vi "PH_ImageStatistician.select Data.vi"(6 "Data Selector":T2 items=["nothing ", "FWHM Major Trace", "FWHM Minor Trace", "Gaussian Fit Order Major Trace", "Gaussian Fit Order Minor Trace", "99% Diameter Major Trace", "99% Diameter Minor Trace", "Theta", "Delta", "Major Diameter", "Minor Diameter", "Azimuth Angle", "Azi Angle rel to Major?", "Ellipticity", "Center of gravity - x", "Center of gravity - y", "Energy"], 8 "Statistician Data":T1) -> (1 "Data chosen?":bool, 2 "Data Legend":string, 3 "Data":dbl)   [LabVIEW 2014, in "PH_ImageStatistician.lvlib"]
doc: "This VI selects the data to be indicated."
uses:
  PH_ImageStatistician.lvlib
  PH_ImageStatistician.select Data.ctl
  PH_ImageStatistician.Statistician Data.ctl
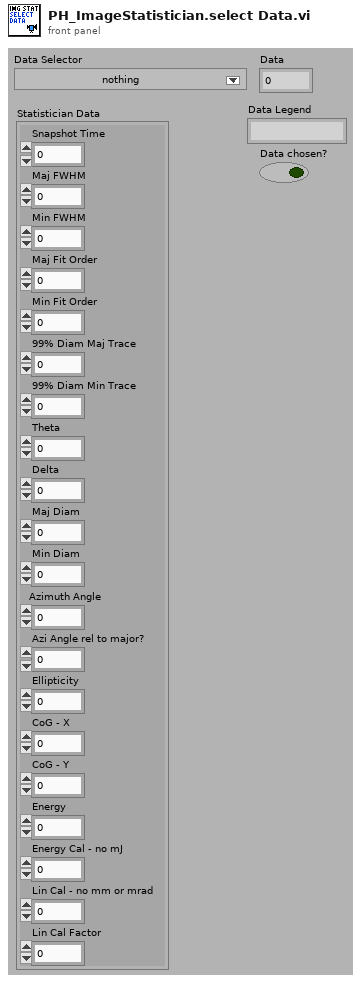
[diagram p1: front panel]
types:
  T1 = typedef "PH_ImageStatistician.lvlib/PH_ImageStatistician.Statistician Data.ctl" = cluster{"Snapshot Time":dbl, "Maj FWHM":dbl, "Min FWHM":dbl, "Maj Fit Order":dbl, "Min Fit Order":dbl, "99% Diam Maj Trace":dbl, "99% Diam Min Trace":dbl, "Theta":dbl, "Delta":dbl, "Maj Diam":dbl, "Min Diam":dbl, "Azimuth Angle":dbl, "Azi Angle rel to major?":dbl, "Ellipticity":dbl, "CoG - X":dbl, "CoG - Y":dbl, "Energy":dbl, "Energy Cal - no mJ":dbl, "Lin Cal - no mm or mrad":dbl, "Lin Cal Factor":dbl}
  T2 = typedef "PH_ImageStatistician.lvlib/PH_ImageStatistician.select Data.ctl" = u16
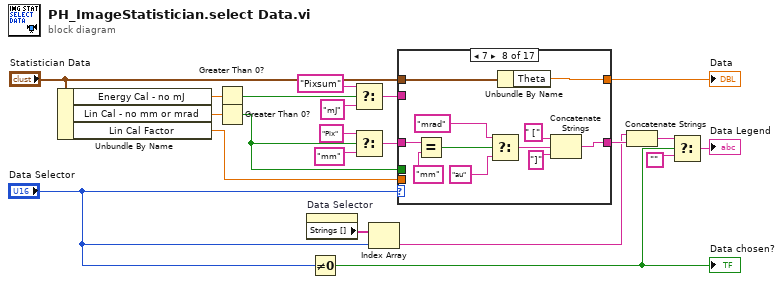
[diagram p0: block diagram]
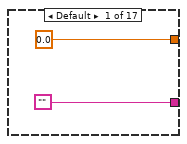
[diagram p2: hidden frame]
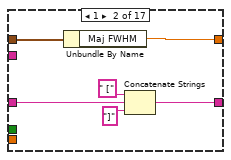
[diagram p3: hidden frame]
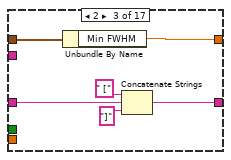
[diagram p4: hidden frame]
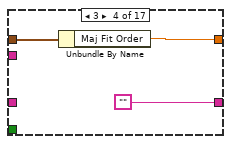
[diagram p5: hidden frame]
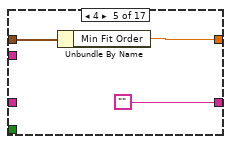
[diagram p6: hidden frame]
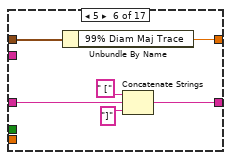
[diagram p7: hidden frame]
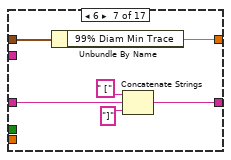
[diagram p8: hidden frame]
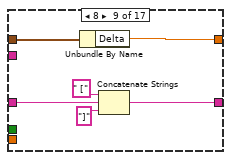
[diagram p9: hidden frame]
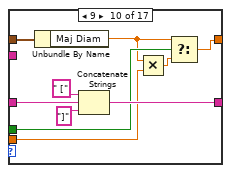
[diagram p10: hidden frame]
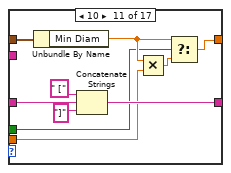
[diagram p11: hidden frame]
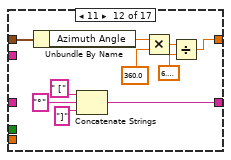
[diagram p12: hidden frame]
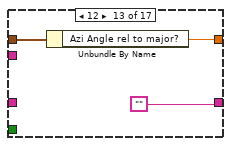
[diagram p13: hidden frame]
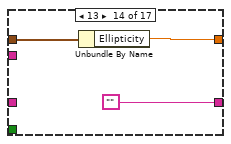
[diagram p14: hidden frame]
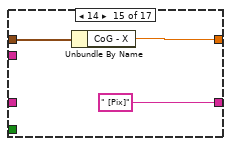
[diagram p15: hidden frame]
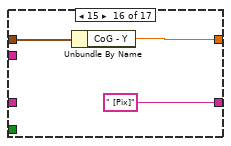
[diagram p16: hidden frame]
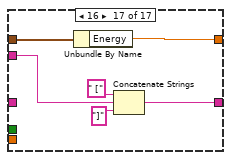
[diagram p17: hidden frame]
diagram:
  n1 = Unbundle By Name("Statistician Data") -> ("Energy Cal - no mJ"=w5:dbl, "Lin Cal - no mm or mrad"=w12:dbl, "Lin Cal Factor"=w8:dbl)
  n2 = Greater Than 0?(x=w5) -> (x > 0?=w4:bool)
  n3 = Greater Than 0?(x=w12) -> (x > 0?=w7:bool)
  n4 = property on="Data Selector" class="Ring (strict)"() -> ("Strings []"=w20:string[])  [unwired: 2 in, 2 out]
  n5 = Not Equal To 0?(x="Data Selector") -> (x != 0?=w17:bool)
  "Data chosen?" <- w17
  n6 = Select(t="Pixsum" ("string"), s=w4, f="mJ") -> (s? t:f=w3:string)
  n7 = Select(t="Pix" ("string"), s=w7, f="mm") -> (s? t:f=w9:string)
  n8 = Index Array(array=w20, index="Data Selector") -> (element=w16:string)
  n9 = case shown="7" "Data Selector" {
    tunnel: [0.0 ("Maj FWHM") w25 w35 w38 w41 w47 w53 w64 w70 w74 w84 w92 w101 w106 w109 w112 w118] -> w21
    tunnel: ["" w28 w32 "" "" w44 w50 w61 w67 w78 w88 w98 "" "" " [Pix]" " [Pix]" w115] -> w18
    tunnel: w9 -> [_ w27 w31 _ _ w43 w49 w60 w66 w77 w87 _ _ _ _ _ _]
    tunnel: w7 -> [_ _ _ _ _ _ _ _ _ w75 w83 _ _ _ _ _ _]
    tunnel: w8 -> [_ _ _ _ _ _ _ _ _ w72 w82 _ _ _ _ _ _]
    tunnel: "Statistician Data" -> [_ w24 w30 w36 w39 w42 w48 w54 w65 w71 w81 w91 w102 w104 w107 w110 w114]
    tunnel: w3 -> [_ _ _ _ _ _ _ _ _ _ _ _ _ _ _ _ w113]
    frame Default {
    }
    frame 1 {
      n10 = Unbundle By Name(w24) -> ("Maj FWHM"=w25:dbl)
      n11 = Concatenate Strings(" [" ("string"), w27, "]" ("string")) -> (w28:string)
    }
    frame 2 {
      n12 = Unbundle By Name(w30) -> ("Min FWHM"=w35:dbl)
      n13 = Concatenate Strings(" [" ("string"), w31, "]" ("string")) -> (w32:string)
    }
    frame 3 {
      n14 = Unbundle By Name(w36) -> ("Maj Fit Order"=w38:dbl)
    }
    frame 4 {
      n15 = Unbundle By Name(w39) -> ("Min Fit Order"=w41:dbl)
    }
    frame 5 {
      n16 = Unbundle By Name(w42) -> ("99% Diam Maj Trace"=w47:dbl)
      n17 = Concatenate Strings(" [" ("string"), w43, "]" ("string")) -> (w44:string)
    }
    frame 6 {
      n18 = Unbundle By Name(w48) -> ("99% Diam Min Trace"=w53:dbl)
      n19 = Concatenate Strings(" [" ("string"), w49, "]" ("string")) -> (w50:string)
    }
    frame 7 {
      n20 = Equal?(x=w60, y="mm") -> (x = y?=w59:bool)
      n21 = Select(t="mrad" ("y"), s=w59, f="au" ("y")) -> (s? t:f=w58:string)
      n22 = Unbundle By Name(w54) -> ("Theta"=w64:dbl)
      n23 = Concatenate Strings(" [" ("string"), w58, "]" ("string")) -> (w61:string)
    }
    frame 8 {
      n24 = Unbundle By Name(w65) -> ("Delta"=w70:dbl)
      n25 = Concatenate Strings(" [" ("string"), w66, "]" ("string")) -> (w67:string)
    }
    frame 9 {
      n26 = Unbundle By Name(w71) -> ("Maj Diam"=w73:dbl)
      n27 = Concatenate Strings(" [" ("string"), w77, "]" ("string")) -> (w78:string)
      n28 = Multiply(x=w73, y=w72) -> (x*y=w76:dbl)
      n29 = Select(t=w73, s=w75, f=w76) -> (s? t:f=w74:dbl)
    }
    frame 10 {
      n30 = Unbundle By Name(w81) -> ("Min Diam"=w85:dbl)
      n31 = Concatenate Strings(" [" ("string"), w87, "]" ("string")) -> (w88:string)
      n32 = Multiply(x=w85, y=w82) -> (x*y=w86:dbl)
      n33 = Select(t=w85, s=w83, f=w86) -> (s? t:f=w84:dbl)
    }
    frame 11 {
      n34 = Unbundle By Name(w91) -> ("Azimuth Angle"=w93:dbl)
      n35 = Concatenate Strings(" [" ("string"), "°", "]" ("string")) -> (w98:string)
      n36 = Multiply(x=w93, y=360.0) -> (x*y=w95:dbl)
      n37 = Divide(x=w95, y=6.283185307179586) -> (x/y=w92:dbl)
    }
    frame 12 {
      n38 = Unbundle By Name(w102) -> ("Azi Angle rel to major?"=w101:dbl)
    }
    frame 13 {
      n39 = Unbundle By Name(w104) -> ("Ellipticity"=w106:dbl)
    }
    frame 14 {
      n40 = Unbundle By Name(w107) -> ("CoG - X"=w109:dbl)
    }
    frame 15 {
      n41 = Unbundle By Name(w110) -> ("CoG - Y"=w112:dbl)
    }
    frame 16 {
      n42 = Unbundle By Name(w114) -> ("Energy"=w118:dbl)
      n43 = Concatenate Strings(" [" ("string"), w113, "]" ("string")) -> (w115:string)
    }
  }
  "Data" <- w21
  n44 = Concatenate Strings(w16, w18) -> (w14:string)
  n45 = Select(t=w14, s=w17, f="") -> (s? t:f=→"Data Legend":string)
